vi "SetUpPanel.vi"(9 "Settings":refnum<vi>) -> ()   [LabVIEW 2015]
uses:
  Ctrls/YesOrNo.ctl
  <vilib>/Utility/sysdir.llb/System Directory Type.ctl
  <vilib>/Utility/config.llb/Write Key (U32).vi
  <vilib>/Utility/config.llb/Write Key (Boolean).vi
  <vilib>/Utility/config.llb/NI_LVConfig.lvlib
panel:
  in  "ConfigTabs":enum32{"UI", "Xset", "Yset", "LineSet"}(tab) caption="AxleConfigTabs"
  in  "Language":u32(ring)=804 caption="Language:" items=["中文"=804, "Engilish"=409]
  in  "ChkUpdatePeriod":u32(ring) caption="检查更新周期:" items=["每个月"=2592000, "每星期"=604800, "每一天"=86400, "每小时"=3600, "每次运行"=1, "从不"=0]
  in  "TimeFormat":u16(ring) caption="时间轴格式" items=["相对时间(秒)", "绝对时间(无日期)", "绝对时间(带日期)"]
  in  "isTimeRerange":T1 caption="时间自动整理"
  in  "isAutoY":T1=TRUE caption="自动Y轴"
  in  "isAutoCurves":T1=TRUE caption="自动配线"
  in  "LineWidthSet":u16(ring) caption="曲线宽度：" items=["0", "1", "2", "3"]
  in  "isShowYValue":T1=TRUE caption="自动显示Y值定义:"
  in  "isShowXY":T1=TRUE caption="浮动显示坐标："
  in  "btnOK":bool
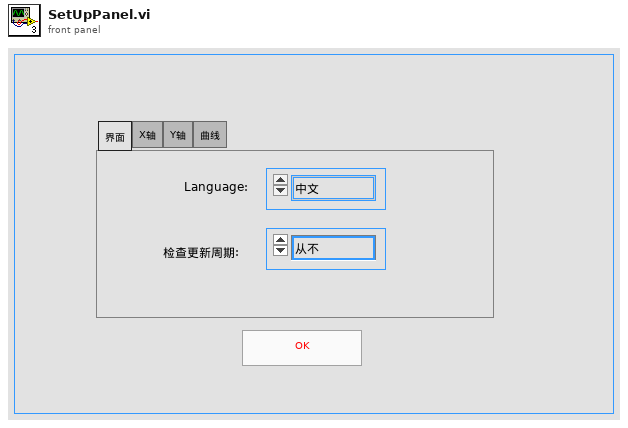
[diagram p1: front panel]
types:
  T1 = typedef "YesOrNo.ctl" = bool
  T2 = typedef "System Directory Type.ctl" = i32
  T3 = typedef "SettingParameters.ctl" = cluster{"LangSet":u32, "TimeFormat":u16, "TimeRerange":bool, "isAutoCurves":bool, "isAutoY":bool, "NeedUpdate":bool, "LastTimChkUpdate":dbl, "NewVersionOnWeb":string, "ChkUpdatePeriod":u32, "LineWidth":u8, "isShowYValue":bool, "isShowXY":bool}
  T4 = typedef "NI_LVConfig.lvlib/Config Data RefNum.ctl" = refnum<k1>
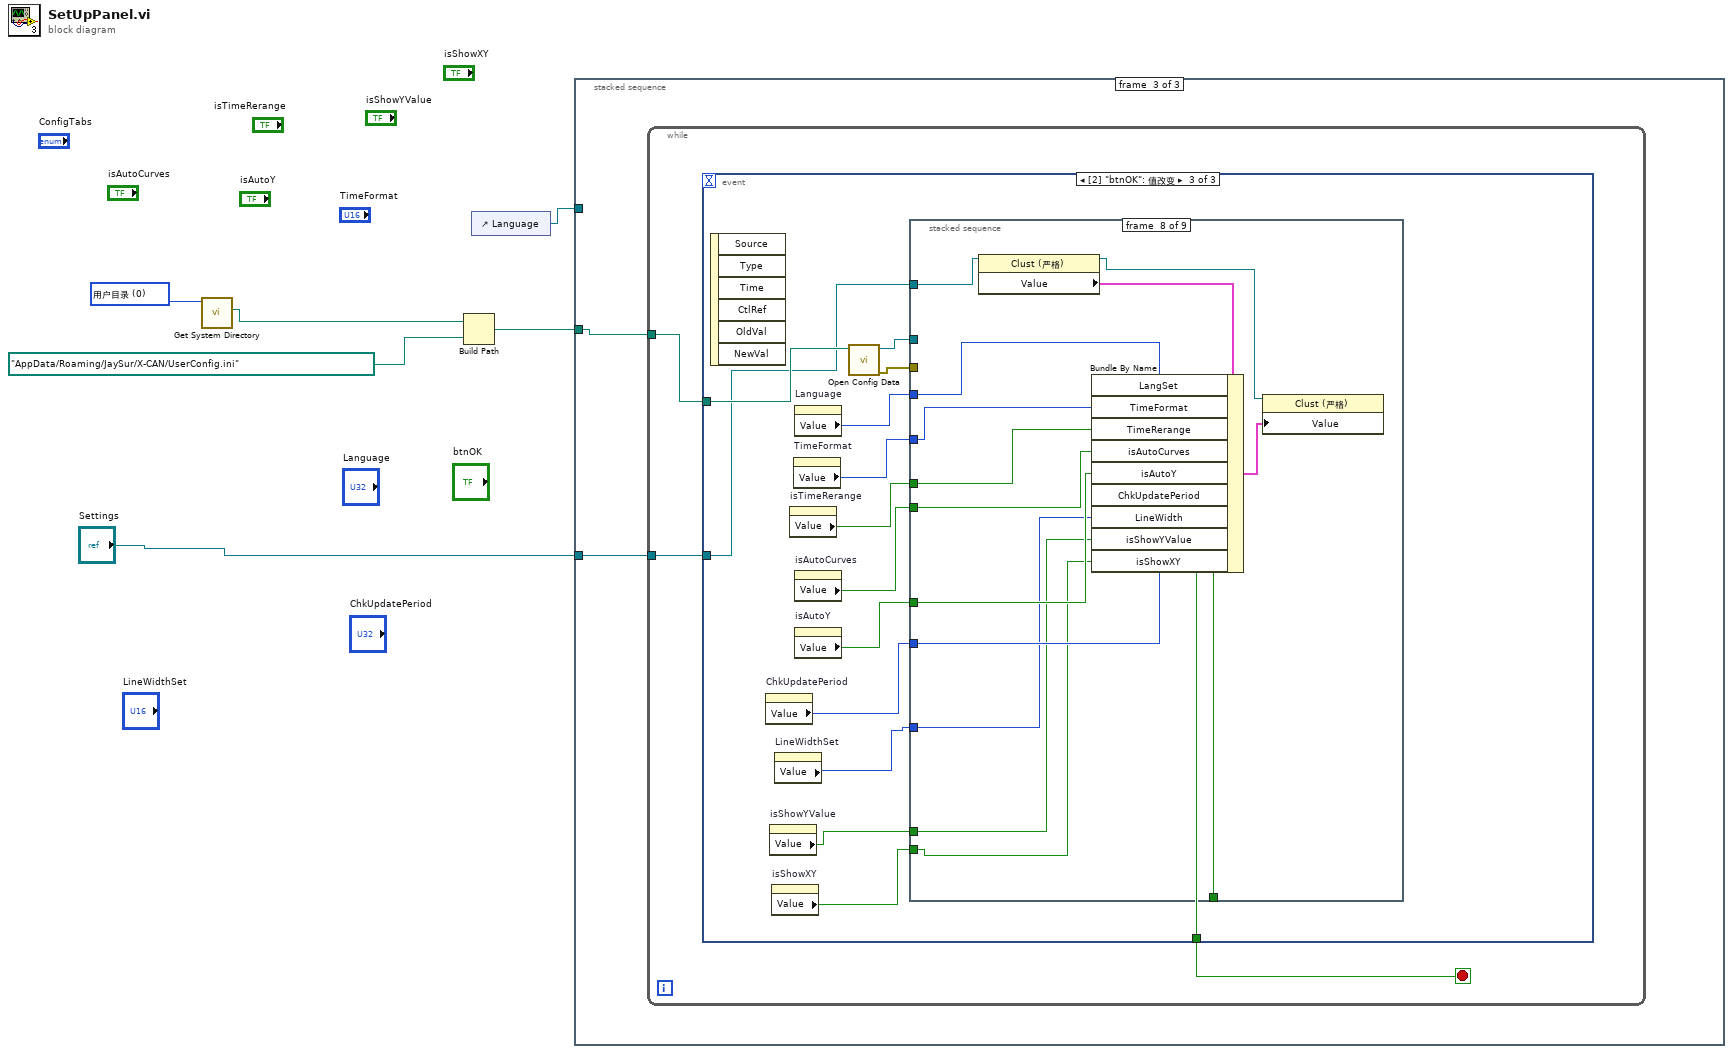
[diagram p0: block diagram]
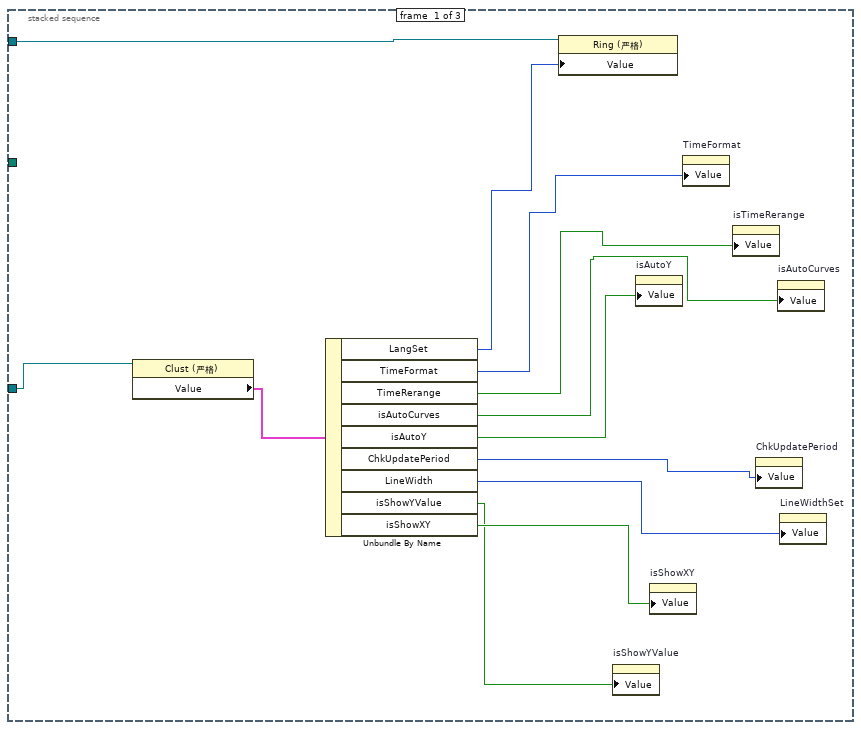
[diagram p2: hidden frame]
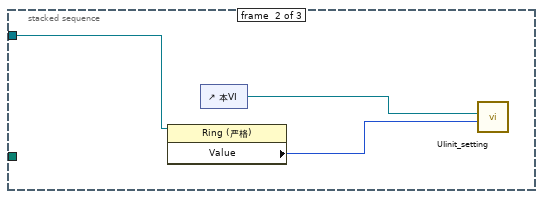
[diagram p3: hidden frame]
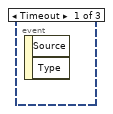
[diagram p4: hidden frame]
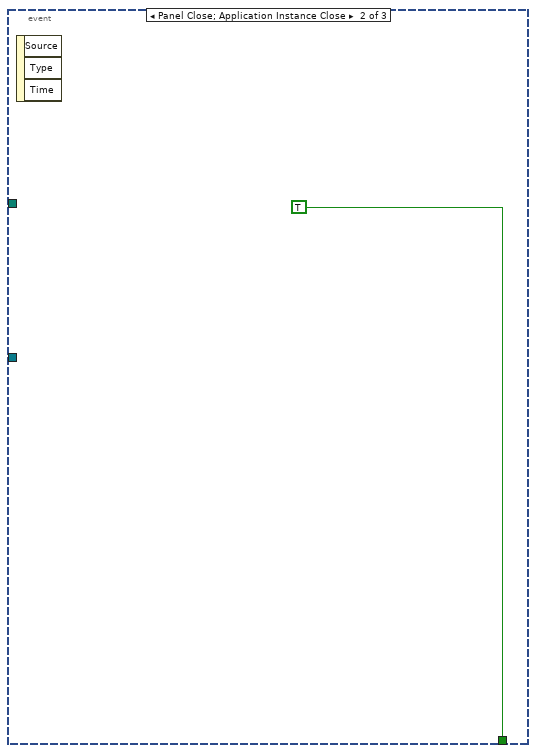
[diagram p5: hidden frame]
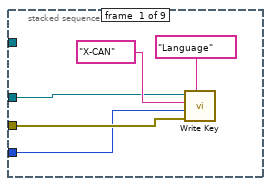
[diagram p6: hidden frame]
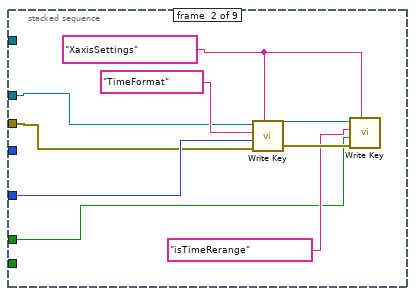
[diagram p7: hidden frame]
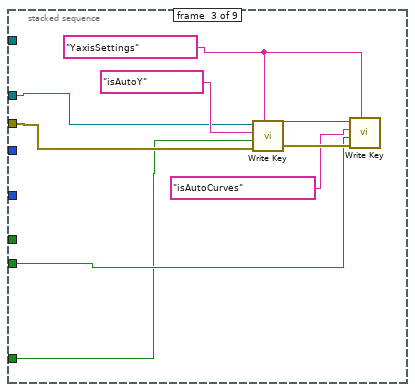
[diagram p8: hidden frame]
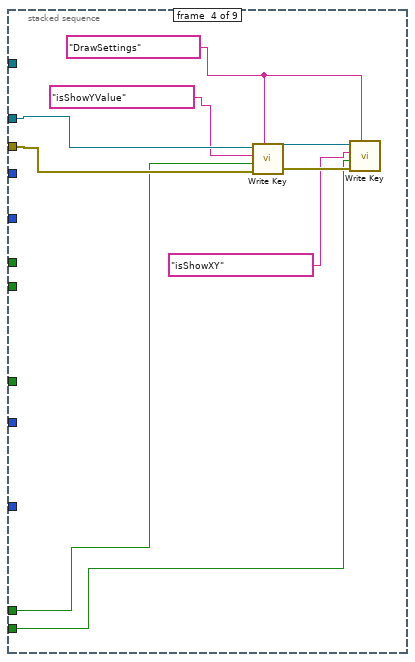
[diagram p9: hidden frame]
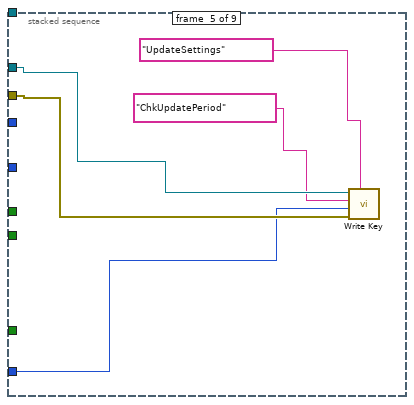
[diagram p10: hidden frame]
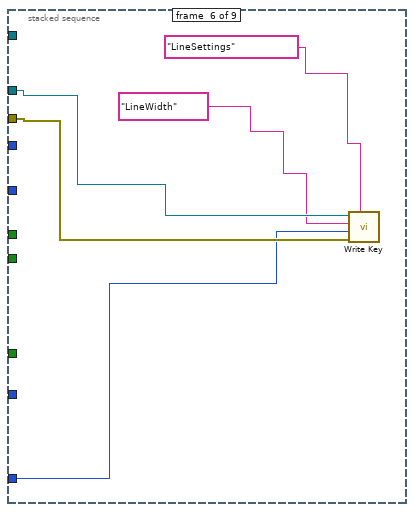
[diagram p11: hidden frame]
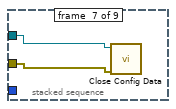
[diagram p12: hidden frame]
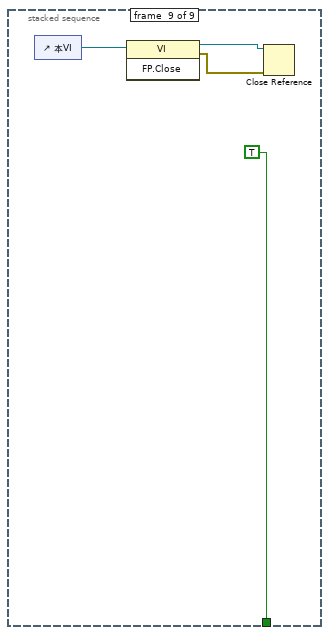
[diagram p13: hidden frame]
diagram:
  w5 = T2 0 items=["用户目录"=0, "用户桌面"=1, "用户文档"=2, "用户应用程序数据"=3, "用户设置"=4, "用户临时目录"=5, "公共文档"=6, "公共应用程序数据"=7, "公共设置"=8, "公共缓存"=13, "系统核心库"=9, "系统安装库"=10, "应用程序文件"=11, "启动盘根目录"=12] ("system directory type")
  n1 = call <vilib>:"Get System Directory.vi"("system directory type"=w5) -> ("system directory"=w4:path)  [unwired: 10 in]
  n2 = Build Path(base path=w4, name or relative path=path "AppData/Roaming/JaySur/X-CAN/UserConfig.ini" ("default name")) -> (appended path=w3:path)
  n3 = control-ref of="Language"() -> (w2:refnum<vi>)
  n4 = stacked-sequence {
    tunnel: w3 -> [_ _ w23]
    tunnel: w2 -> [w18 w20 _]
    tunnel: "Settings" -> [w17 _ w22]
    frame #0 {
      n5 = property class="Clust (严格)"(reference=w17) -> ("Value"=w16:T3)  [unwired: 1 in, 2 out]
      n6 = Unbundle By Name(w16) -> ("LangSet"=w11:u32, "TimeFormat"=w12:u16, "TimeRerange"=w13:bool, "isAutoCurves"=w14:bool, "isAutoY"=w15:bool, "ChkUpdatePeriod"=w10:u32, "LineWidth"=w9:u8, "isShowYValue"=w7:bool, "isShowXY"=w8:bool)
      n7 = property class="Ring (严格)"(reference=w18, "Value"=w11) -> ()  [unwired: 1 in, 2 out]
      n8 = property on="isShowYValue" class="Bool (严格)"("Value"=w7) -> ()  [unwired: 2 in, 2 out]
      n9 = property on="isAutoY" class="Bool (严格)"("Value"=w15) -> ()  [unwired: 2 in, 2 out]
      n10 = property on="isShowXY" class="Bool (严格)"("Value"=w8) -> ()  [unwired: 2 in, 2 out]
      n11 = property on="TimeFormat" class="Ring (严格)"("Value"=w12) -> ()  [unwired: 2 in, 2 out]
      n12 = property on="isTimeRerange" class="Bool (严格)"("Value"=w13) -> ()  [unwired: 2 in, 2 out]
      n13 = property on="ChkUpdatePeriod" class="Ring (严格)"("Value"=w10) -> ()  [unwired: 2 in, 2 out]
      n14 = property on="isAutoCurves" class="Bool (严格)"("Value"=w14) -> ()  [unwired: 2 in, 2 out]
      n15 = property on="LineWidthSet" class="Ring (严格)"("Value"=w9) -> ()  [unwired: 2 in, 2 out]
    }
    frame #1 {
      n16 = property class="Ring (严格)"(reference=w20) -> ("Value"=w19:u32)  [unwired: 1 in, 2 out]
      n17 = control-ref of="本VI"() -> (w21:refnum<vi>)
      n18 = call "UIinit_setting.vi"("Language"=w19, "VIref"=w21) -> ()  [unwired: 10 in]
    }
    frame #2 {
      n19 = while {
        tunnel: w23 -> [w26]
        tunnel: w22 -> [w24]
        stop <- w25 stop-if-true
        n20 = event shown="[2] \"btnOK\": 值改变" {
          selector: _ -> [_ _ _]
          dyn-events: _ -> [_ _ _]
          timeout: _ -> [_ _ _]
          tunnel: w26 -> [_ _ w38]
          tunnel: [_ TRUE w41] -> w25
          tunnel: w24 -> [_ _ w32]
          event Timeout {
            n21 = event-data() -> ()  [unwired: 1 in, 2 out]
          }
          event Panel Close; Application Instance Close {
            n22 = event-data() -> ()  [unwired: 1 in, 3 out]
          }
          event "btnOK": Value Change {
            n23 = event-data() -> ()  [unwired: 1 in, 6 out]
            n24 = property on="ChkUpdatePeriod" class="Ring (严格)"() -> ("Value"=w31:u32)  [unwired: 2 in, 2 out]
            n25 = property on="isShowYValue" class="Bool (严格)"() -> ("Value"=w28:T1)  [unwired: 2 in, 2 out]
            n26 = property on="isShowXY" class="Bool (严格)"() -> ("Value"=w29:T1)  [unwired: 2 in, 2 out]
            n27 = property on="LineWidthSet" class="Ring (严格)"() -> ("Value"=w30:u16)  [unwired: 2 in, 2 out]
            n28 = property on="isTimeRerange" class="Bool (严格)"() -> ("Value"=w35:T1)  [unwired: 2 in, 2 out]
            n29 = property on="TimeFormat" class="Ring (严格)"() -> ("Value"=w34:u16)  [unwired: 2 in, 2 out]
            n30 = property on="Language" class="Ring (严格)"() -> ("Value"=w33:u32)  [unwired: 2 in, 2 out]
            n31 = property on="isAutoCurves" class="Bool (严格)"() -> ("Value"=w36:T1)  [unwired: 2 in, 2 out]
            n32 = property on="isAutoY" class="Bool (严格)"() -> ("Value"=w37:T1)  [unwired: 2 in, 2 out]
            n33 = call <vilib>:"Open Config Data.vi"("configuration file path"=w38) -> ("error out"=w39:errorcluster, "refnum"=w40:T4)  [unwired: 8 in, 1 out]
            n34 = stacked-sequence {
              tunnel: [_ _ _ _ _ _ _ _ TRUE] -> w41
              tunnel: w40 -> [w44 w53 w63 w73 w78 w83 w85 _ _]
              tunnel: w39 -> [w43 w52 w62 w72 w77 w82 w84 _ _]
              tunnel: w37 -> [_ _ w56 _ _ _ _ w95 _]
              tunnel: w36 -> [_ _ w57 _ _ _ _ w94 _]
              tunnel: w35 -> [_ w47 _ _ _ _ _ w93 _]
              tunnel: w34 -> [_ w54 _ _ _ _ _ w92 _]
              tunnel: w33 -> [w42 _ _ _ _ _ _ w91 _]
              tunnel: w32 -> [_ _ _ _ _ _ _ w90 _]
              tunnel: w31 -> [_ _ _ _ w76 _ _ w89 _]
              tunnel: w30 -> [_ _ _ _ _ w81 _ w88 _]
              tunnel: w29 -> [_ _ _ w69 _ _ _ w86 _]
              tunnel: w28 -> [_ _ _ w68 _ _ _ w87 _]
              frame #0 {
                n35 = call-poly <vilib>:"Write Key.vi"("section"="Language", "error in (no error)"=w43, "value"=w42, "key"="X-CAN", "refnum"=w44) -> ()  [unwired: 4 in, 3 out]
              }
              frame #1 {
                w51 = "XaxisSettings" ("section")
                n36 = call-poly <vilib>:"Write Key.vi"("section"=w51, "error in (no error)"=w52, "value"=w54, "key"="TimeFormat", "refnum"=w53) -> ("error out"=w49:errorcluster, "refnum out"=w50:T4)  [unwired: 4 in, 1 out]
                n37 = call-poly <vilib>:"Write Key.vi"("section"=w51, "error in (no error)"=w49, "value"=w47, "key"="isTimeRerange", "refnum"=w50) -> ()  [unwired: 4 in, 3 out]
              }
              frame #2 {
                w61 = "YaxisSettings" ("section")
                n38 = call-poly <vilib>:"Write Key.vi"("section"=w61, "error in (no error)"=w62, "value"=w56, "key"="isAutoY", "refnum"=w63) -> ("error out"=w59:errorcluster, "refnum out"=w60:T4)  [unwired: 4 in, 1 out]
                n39 = call-poly <vilib>:"Write Key.vi"("section"=w61, "error in (no error)"=w59, "value"=w57, "key"="isAutoCurves", "refnum"=w60) -> ()  [unwired: 4 in, 3 out]
              }
              frame #3 {
                w67 = "DrawSettings" ("section")
                n40 = call-poly <vilib>:"Write Key.vi"("section"=w67, "error in (no error)"=w72, "value"=w68, "key"="isShowYValue", "refnum"=w73) -> ("error out"=w70:errorcluster, "refnum out"=w71:T4)  [unwired: 4 in, 1 out]
                n41 = call-poly <vilib>:"Write Key.vi"("section"=w67, "error in (no error)"=w70, "value"=w69, "key"="isShowXY", "refnum"=w71) -> ()  [unwired: 4 in, 3 out]
              }
              frame #4 {
                n42 = call-poly <vilib>:"Write Key.vi"("section"="UpdateSettings", "error in (no error)"=w77, "value"=w76, "key"="ChkUpdatePeriod", "refnum"=w78) -> ()  [unwired: 4 in, 3 out]
              }
              frame #5 {
                n43 = call-poly <vilib>:"Write Key.vi"("section"="LineSettings", "error in (no error)"=w82, "value"=w81, "key"="LineWidth", "refnum"=w83) -> ()  [unwired: 4 in, 3 out]
              }
              frame #6 {
                n44 = call <vilib>:"Close Config Data.vi"("error in (no error)"=w84, "refnum"=w85) -> ()  [unwired: 8 in, 2 out]
              }
              frame #7 {
                n45 = property class="Clust (严格)"(reference=w90) -> (reference out=w97:refnum<vi>, "Value"=w98:T3)  [unwired: 1 in, 1 out]
                n46 = Bundle By Name(cluster=w98, "LangSet"=w91, "TimeFormat"=w92, "TimeRerange"=w93, "isAutoCurves"=w94, "isAutoY"=w95, "ChkUpdatePeriod"=w89, "LineWidth"=w88, "isShowYValue"=w87, "isShowXY"=w86) -> (w96:T3)
                n47 = property class="Clust (严格)"(reference=w97, "Value"=w96) -> ()  [unwired: 1 in, 2 out]
              }
              frame #8 {
                n48 = control-ref of="本VI"() -> (w101:refnum<vi>)
                n49 = invoke class="VI" method="FP.Close"(reference=w101) -> (reference out=w100:refnum<vi>, error out=w99:errorcluster)  [unwired: 2 in, 1 out]
                n50 = Close Reference(reference=w100, error in (no error)=w99) -> ()  [unwired: 1 out]
              }
            }
          }
        }
      }
    }
  }
